vi "StringList2StringArray.vi"(1 "Active Channel Numbers String":string) -> (0 "Array":string[](array[string]))   [LabVIEW 2019]
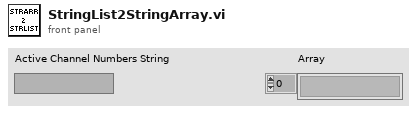
[diagram p1: front panel]
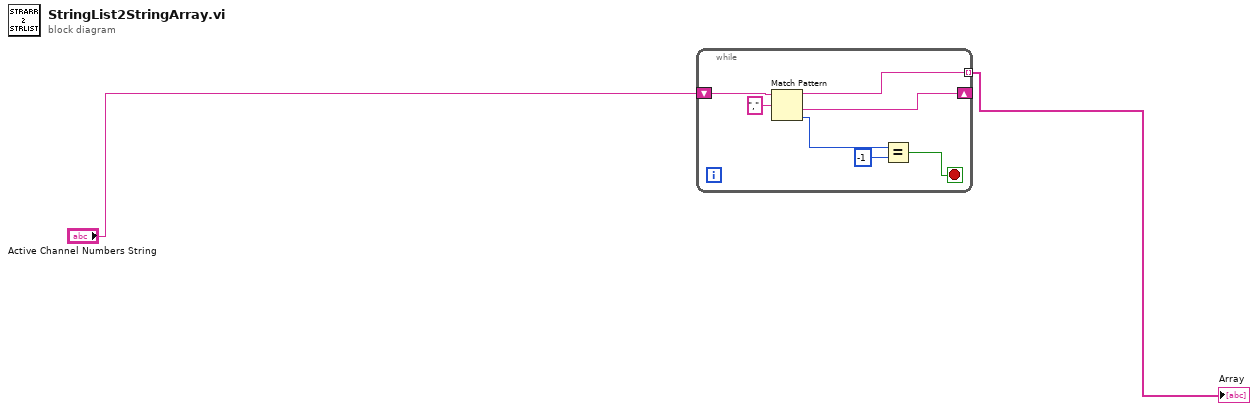
[diagram p0: block diagram]
diagram:
  n1 = while {
    tunnel: [w7] -> w2 mode=indexing
    shift-right: [w6] -> _
    shift-left: "Active Channel Numbers String" -> [w9]
    stop <- w3 stop-if-true
    n2 = Match Pattern(string=w9, regular expression=",") -> (before substring=w7:string, after substring=w6:string, offset past match=w5:i32)  [unwired: 1 in, 1 out]
    n3 = Equal?(x=w5, y=-1) -> (x = y?=w3:bool)
  }
  "Array" <- w2
